vi "Draw Multiline Text At Point.vi"(0 "text orientation":T1(ring), 4 "BG color(transparent)":u32(colorbox)=16777216, 5 "[user-specified font]":T5={"Font Name:"="", "Size"=12, "Strikeout?"=FALSE, "Italic?"=FALSE, "Underline?"=FALSE, "Outline?"=FALSE, "Shadow?"=FALSE, "Bold?"=FALSE}, 6 "text color(black)":u32(colorbox), 7 "desired font(Application)":T4(ring)=enum."Application Font", 8 "text":string, 9 "alignment(left, top,text)":T3, 10 "origin":cluster{"x":i16, "y":i16}, 11 "picture":picture) -> (2 "text rect":T2, 3 "new picture":picture)   [LabVIEW 2024, in "Controller.lvlib" / "Controller.lvclass"]
doc: "Draws a string into a picture.\n\nWiebe Walstra\nwww.carya.nl"
uses:
  Controller/Controller/Controller.lvclass
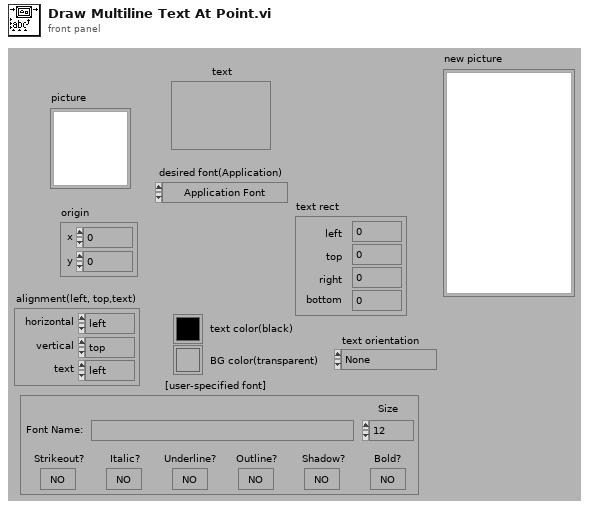
[diagram p1: front panel]
types:
  T1 = enum16{"None", "Stacked", "Clockwise", "Counterclockwise"}
  T2 = cluster{"left":i16, "top":i16, "right":i16, "bottom":i16}
  T3 = cluster{"horizontal":enum16{"left", "center", "right"}, "vertical":enum16{"top", "center", "bottom"}, "text":enum16{"left", "center", "right"}}
  T4 = enum16{"User-specified Font", "Application Font", "System Font", "Dialog Font"}
  T5 = cluster{"Font Name:":string, "Size":i16, "Strikeout?":bool, "Italic?":bool, "Underline?":bool, "Outline?":bool, "Shadow?":bool, "Bold?":bool}
  T6 = cluster{"horizontal":enum16{"left", "center", "right"}, "vertical":enum16{"top", "center", "bottom"}}
  T7 = cluster{"Strikeout?":bool, "Italic?":bool, "Underline?":bool, "Outline?":bool, "Shadow?":bool}
  T8 = cluster{"opcode - NewFont":i16, i32, i8, "platform":i8, "Size":i16, i16, i16}
  T9 = cluster{i32, "text color(black)":u32, "BG color(transparent)":u32, "Black":u32, "White":u32}
  T10 = cluster{"top":i16, "left":i16, "bottom":i16, "right":i16}
  T11 = cluster{"opcode - TBox":i16, i32, i32, cluster{"top":i16, "left":i16, "bottom":i16, "right":i16}, i32}
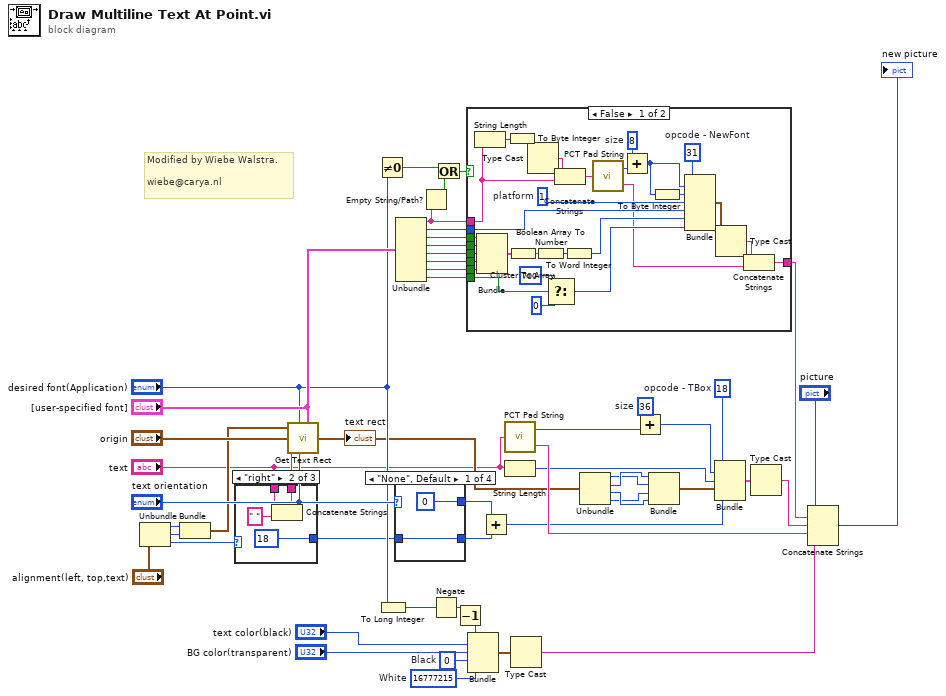
[diagram p0: block diagram]
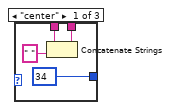
[diagram p2: hidden frame]
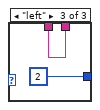
[diagram p3: hidden frame]
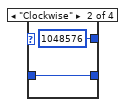
[diagram p4: hidden frame]
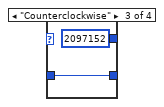
[diagram p5: hidden frame]
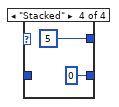
[diagram p6: hidden frame]
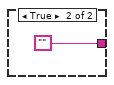
[diagram p7: hidden frame]
diagram:
  w36 = u32 0  # Black
  w37 = u32 16777215  # White
  w24 = 36  # size
  w21 = i16 18  # opcode - TBox
  # "Modified by Wiebe Walstra.\n\nwiebe@carya.nl"
  n1 = Unbundle("alignment(left, top,text)") -> ("horizontal"=w10:enum16{"left", "center", "right"}, "vertical"=w9:enum16{"top", "center", "bottom"}, "text"=w7:enum16{"left", "center", "right"})
  n2 = Bundle("horizontal"=w10, "vertical"=w9) -> (w8:T6)  [unwired: 1 in]
  n3 = case shown="\"right\"" w7 {
    tunnel: [34 18 2] -> w6
    tunnel: [w54 w57 w61] -> w2
    tunnel: "text" -> [w55 w58 w61]
    frame "center" {
      n4 = Concatenate Strings(w55, " " ("string")) -> (w54:string)
    }
    frame "right" {
      n5 = Concatenate Strings(w58, " " ("string")) -> (w57:string)
    }
    frame "left" {
    }
  }
  n6 = call <vilib>:"Get Text Rect.vi"("alignment(left, top)"=w8, "desired font(Application)"="desired font(Application)", "origin(0,0)"="origin", "text"=w2, "text orientation"="text orientation", "[user-specified font]"="[user-specified font]") -> ("rect"=w13:T2)  [unwired: 3 in]
  "text rect" <- w13
  n7 = Not Equal To 0?(x="desired font(Application)") -> (x != 0?=w46:bool)
  n8 = To Long Integer(number="desired font(Application)") -> (32bit integer=w52:i32)
  n9 = case shown="\"None\", Default" "text orientation" {
    tunnel: [0 1048576 2097152 5] -> w3
    tunnel: [w63 w65 w67 0] -> w5
    tunnel: w6 -> [w63 w65 w67 _]
    frame "None", Default {
    }
    frame "Clockwise" {
    }
    frame "Counterclockwise" {
    }
    frame "Stacked" {
    }
  }
  n10 = Unbundle("[user-specified font]") -> ("Font Name:"=w27:string, "Size"=w28:i16, "Strikeout?"=w38:bool, "Italic?"=w39:bool, "Underline?"=w40:bool, "Outline?"=w41:bool, "Shadow?"=w42:bool, "Bold?"=w43:bool)
  n11 = Empty String/Path?(string/path=w27) -> (empty?=w44:bool)
  n12 = Negate(x=w52) -> (-x=w29:i32)
  n13 = Or(x=w46, y=w44) -> (x .or. y?=w45:bool)
  n14 = Decrement(x=w29) -> (x-1=w30:i32)
  n15 = case shown="False" w45 {
    tunnel: w27 -> [w75 _]
    tunnel: w28 -> [w90 _]
    tunnel: w38 -> [w83 _]
    tunnel: w39 -> [w84 _]
    tunnel: w40 -> [w89 _]
    tunnel: w41 -> [w88 _]
    tunnel: w42 -> [w87 _]
    tunnel: w43 -> [w86 _]
    tunnel: [w71 ""] -> w51
    frame False {
      w93 = i8 1  # platform
      w98 = 8  # size
      w92 = i16 31  # opcode - NewFont
      n16 = String Length(string=w75) -> (length=w77:i32)
      n17 = Bundle("Strikeout?"=w83, "Italic?"=w84, "Underline?"=w89, "Outline?"=w88, "Shadow?"=w87) -> (w85:T7)  [unwired: 1 in]
      n18 = To Byte Integer(number=w77) -> (8bit integer=w76:i8)
      n19 = Cluster To Array(cluster=w85) -> (array=w82:bool[])
      n20 = Type Cast(x=w76) -> (*(type *) &x=w78:string)  [unwired: 1 in]
      n21 = Boolean Array To Number(Boolean array=w82) -> (number=w81:u32)
      n22 = Select(t=i16 700, s=w86, f=i16 0) -> (s? t:f=w97:i16)
      n23 = Concatenate Strings(w78, w75) -> (w74:string)
      n24 = To Word Integer(number=w81) -> (16bit integer=w80:i16)
      n25 = call <vilib>:"PCT Pad String.vi"("string"=w74) -> ("padded length"=w99:i32, "padded string"=w72:string)
      n26 = Add(x=w98, y=w99) -> (x+y=w91:i32)
      n27 = To Byte Integer(number=w91) -> (8bit integer=w79:i8)
      n28 = Bundle("opcode - NewFont"=w92, w91, w79, "platform"=w93, "Size"=w90, w80, w97) -> (w94:T8)  [unwired: 1 in]
      n29 = Type Cast(x=w94) -> (*(type *) &x=w73:string)  [unwired: 1 in]
      n30 = Concatenate Strings(w73, w72) -> (w71:string)
    }
    frame True {
    }
  }
  n31 = Bundle(w30, "text color(black)"="text color(black)", "BG color(transparent)"="BG color(transparent)", "Black"=w36, "White"=w37) -> (w23:T9)  [unwired: 1 in]
  n32 = Add(x=w3, y=w5) -> (x+y=w4:i32)
  n33 = call <vilib>:"PCT Pad String.vi"("string"="text") -> ("padded length"=w47:i32, "padded string"=w49:string)
  n34 = String Length(string="text") -> (length=w25:i32)
  n35 = Type Cast(x=w23) -> (*(type *) &x=w48:string)  [unwired: 1 in]
  n36 = Unbundle(w13) -> ("left"=w31:i16, "top"=w32:i16, "right"=w34:i16, "bottom"=w33:i16)
  n37 = Add(x=w24, y=w47) -> (x+y=w26:i32)
  n38 = Bundle("top"=w32, "left"=w31, "bottom"=w33, "right"=w34) -> (w35:T10)  [unwired: 1 in]
  n39 = Bundle("opcode - TBox"=w21, w26, w25, w35, w4) -> (w22:T11)  [unwired: 1 in]
  n40 = Type Cast(x=w22) -> (*(type *) &x=w50:string)  [unwired: 1 in]
  n41 = Concatenate Strings("picture", w51, w50, w49, w48) -> (→"new picture":picture)
